vi "expo drive.vi"(1 "Expo":dbl, 2 "Raw Input":dbl) -> (0 "Output":dbl)   [LabVIEW 2014]
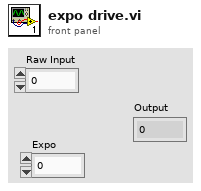
[diagram p1: front panel]
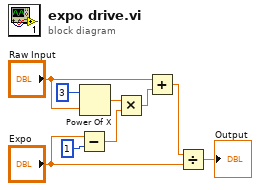
[diagram p0: block diagram]
diagram:
  n1 = Subtract(x="Expo", y=1) -> (x-y=w6:dbl)
  n2 = Power Of X(1:"Raw Input", 2:3) -> (0:w7:dbl)
  n3 = Multiply(x=w7, y=w6) -> (x*y=w5:dbl)
  n4 = Add(x="Raw Input", y=w5) -> (x+y=w3:dbl)
  n5 = Divide(x=w3, y="Expo") -> (x/y=→"Output":dbl)
